vi "Handle Status Code.vi"(8 "error in":errorcluster, 10 "TPCANHandle":T1=81 items=["PCAN_NONEBUS"=0, "PCAN_USBBUS1"=81, "PCAN_USBBUS2"=82, "PCAN_USBBUS3"=83, "PCAN_USBBUS4"=84, "PCAN_USBBUS5"=85, "PCAN_USBBUS6"=86, "PCAN_USBBUS7"=87, "PCAN_USBBUS8"=88, "PCAN_USBBUS9"=1289, "PCAN_USBBUS10"=1290, "PCAN_USBBUS11"=1291, "PCAN_USBBUS12"=1292, "PCAN_USBBUS13"=1293, "PCAN_USBBUS14"=1294, "PCAN_USBBUS15"=1295, "PCAN_USBBUS16"=1296], 11 "TPCANStatus":T2 items=["PCAN_ERROR_OK"=0, "PCAN_ERROR_XMTFULL"=1, "PCAN_ERROR_OVERRUN"=2, "PCAN_ERROR_BUSLIGHT"=4, "PCAN_ERROR_BUSHEAVY"=8, "PCAN_ERROR_BUSPASSIVE"=262144, "PCAN_ERROR_BUSOFF"=16, "PCAN_ERROR_QRCVEMPTY"=32, "PCAN_ERROR_QOVERRUN"=64, "PCAN_ERROR_QXMTFULL"=128, "PCAN_ERROR_REGTEST"=256, "PCAN_ERROR_NODRIVER"=512, "PCAN_ERROR_HWINUSE"=1024, "PCAN_ERROR_NETINUSE"=2048, "PCAN_ERROR_ILLHW"=5120, "PCAN_ERROR_ILLNET"=6144, "PCAN_ERROR_ILLCLIENT"=7168, "PCAN_ERROR_RESOURCE"=8192, "PCAN_ERROR_ILLPARAMTYPE"=16384, "PCAN_ERROR_ILLPARAMVAL"=32768, "PCAN_ERROR_UNKNOWN"=65536, "PCAN_ERROR_ILLDATA"=131072, "PCAN_ERROR_ILLMODE"=524288, "PCAN_ERROR_CAUTION"=33554432, "PCAN_ERROR_INITIALIZE"=67108864, "PCAN_ERROR_ILLOPERATION"=134217728]) -> (0 "error out":errorcluster)   [LabVIEW 2018, in "PCANBasic.lvlib"]
uses:
  PCANBasic.lvlib
  TPCANStatus.ctl
  TPCANHandle.ctl
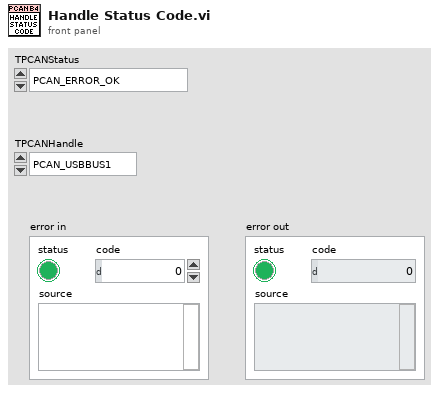
[diagram p1: front panel]
types:
  T1 = typedef "PCANBasic.lvlib/TPCANHandle.ctl" = u16
  T2 = typedef "PCANBasic.lvlib/TPCANStatus.ctl" = u32
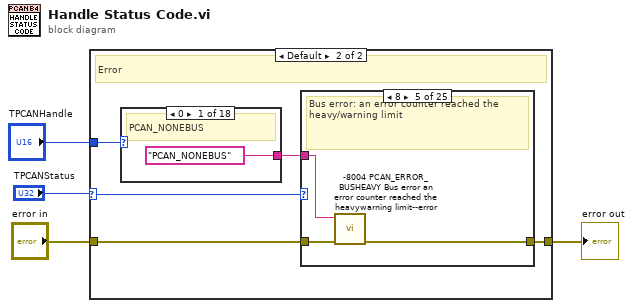
[diagram p0: block diagram]
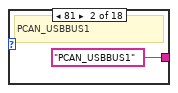
[diagram p3: hidden frame]
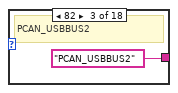
[diagram p4: hidden frame]
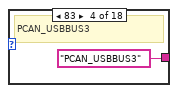
[diagram p5: hidden frame]
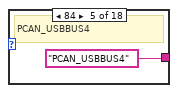
[diagram p6: hidden frame]
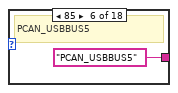
[diagram p7: hidden frame]
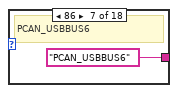
[diagram p8: hidden frame]
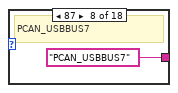
[diagram p9: hidden frame]
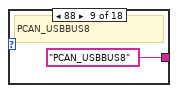
[diagram p10: hidden frame]
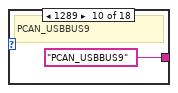
[diagram p11: hidden frame]
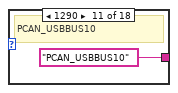
[diagram p12: hidden frame]
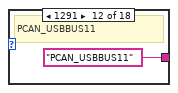
[diagram p13: hidden frame]
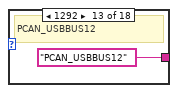
[diagram p14: hidden frame]
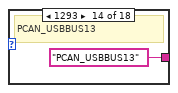
[diagram p15: hidden frame]
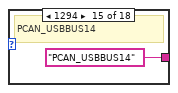
[diagram p16: hidden frame]
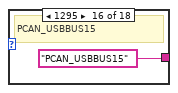
[diagram p17: hidden frame]
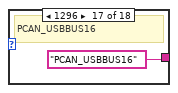
[diagram p18: hidden frame]
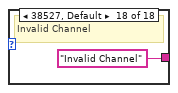
[diagram p19: hidden frame]
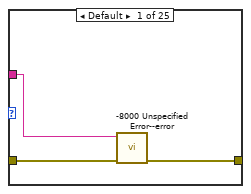
[diagram p20: hidden frame]
diagram:
  n1 = case shown="Default" "TPCANStatus" {
    selector: "TPCANStatus" -> [_ w10]
    tunnel: [w5 w8] -> w4
    tunnel: "error in" -> [w5 w9]
    tunnel: "TPCANHandle" -> [_ w7]
    frame 0 {
      # "OK"
    }
    frame Default {
      # "Error"
      n2 = case shown="0" w7 {
        tunnel: ["PCAN_NONEBUS" "PCAN_USBBUS1" "PCAN_USBBUS2" "PCAN_USBBUS3" "PCAN_USBBUS4" "PCAN_USBBUS5" "PCAN_USBBUS6" "PCAN_USBBUS7" "PCAN_USBBUS8" "PCAN_USBBUS9" "PCAN_USBBUS10" "PCAN_USBBUS11" "PCAN_USBBUS12" "PCAN_USBBUS13" "PCAN_USBBUS14" "PCAN_USBBUS15" "PCAN_USBBUS16" "Invalid Channel"] -> w6
        frame 0 {
          # "PCAN_NONEBUS"
        }
        frame 81 {
          # "PCAN_USBBUS1"
        }
        frame 82 {
          # "PCAN_USBBUS2"
        }
        frame 83 {
          # "PCAN_USBBUS3"
        }
        frame 84 {
          # "PCAN_USBBUS4"
        }
        frame 85 {
          # "PCAN_USBBUS5"
        }
        frame 86 {
          # "PCAN_USBBUS6"
        }
        frame 87 {
          # "PCAN_USBBUS7"
        }
        frame 88 {
          # "PCAN_USBBUS8"
        }
        frame 1289 {
          # "PCAN_USBBUS9"
        }
        frame 1290 {
          # "PCAN_USBBUS10"
        }
        frame 1291 {
          # "PCAN_USBBUS11"
        }
        frame 1292 {
          # "PCAN_USBBUS12"
        }
        frame 1293 {
          # "PCAN_USBBUS13"
        }
        frame 1294 {
          # "PCAN_USBBUS14"
        }
        frame 1295 {
          # "PCAN_USBBUS15"
        }
        frame 1296 {
          # "PCAN_USBBUS16"
        }
        frame 38527, Default {
          # "Invalid Channel"
        }
      }
      n3 = case shown="8" w10 {
        tunnel: w9 -> [w31 w34 w37 w40 w43 w46 w49 w52 w55 w58 w61 w64 w67 w70 w73 w76 w79 w82 w85 w88 w91 w94 w96 w100 w103]
        tunnel: [w30 w33 w36 w39 w42 w45 w48 w51 w54 w57 w60 w63 w66 w69 w72 w75 w78 w81 w84 w87 w90 w93 w97 w99 w102] -> w8
        tunnel: w6 -> [w29 w32 w35 w38 w41 w44 w47 w50 w53 w56 w59 w62 w65 w68 w71 w74 w77 w80 w83 w86 w89 w92 w95 w98 w101]
        frame Default {
          n4 = call "-8000 Unspecified Error--error.vi"("error in"=w31, "Argument"=w29) -> ("error out"=w30:errorcluster)  [unwired: 8 in, 1 out]
        }
        frame 1 {
          # "Transmit buffer in CAN controller is full"
          n5 = call "-8001 PCAN_ERROR_XMTFULL Transmit buffer in CAN controller is full--error.vi"("error in"=w34, "Channel"=w32) -> ("error out"=w33:errorcluster)  [unwired: 8 in, 1 out]
        }
        frame 2 {
          # "CAN Controller was read too late"
          n6 = call "-8002 PCAN_ERROR_OVERRUN CAN Controller was read too late--error.vi"("error in"=w37, "Channel"=w35) -> ("error out"=w36:errorcluster)  [unwired: 8 in, 1 out]
        }
        frame 4 {
          # "Bus error: an error counter reached the 'light' limit"
          n7 = call "-8003 PCAN_ERROR_BUSLIGHT Bus error an error counter reached the 'light' limit--error.vi"("error in"=w40, "Channel"=w38) -> ("error out"=w39:errorcluster)  [unwired: 8 in, 1 out]
        }
        frame 8 {
          # "Bus error: an error counter reached the heavy/warning limit"
          n8 = call "-8004 PCAN_ERROR_BUSHEAVY Bus error an error counter reached the heavywarning limit--error.vi"("error in"=w43, "Channel"=w41) -> ("error out"=w42:errorcluster)  [unwired: 8 in, 1 out]
        }
        frame 16 {
          # "Bus error: the CAN controller is in bus-off state"
          n9 = call "-8005 PCAN_ERROR_BUSOFF Bus error the CAN controller is in bus-off state--error.vi"("error in"=w46, "Channel"=w44) -> ("error out"=w45:errorcluster)  [unwired: 8 in, 1 out]
        }
        frame 32 {
          # "Receive queue is empty"
          n10 = call "-8006 PCAN_ERROR_QRCVEMPTY Receive queue is empty--error.vi"("error in"=w49, "Channel"=w47) -> ("error out"=w48:errorcluster)  [unwired: 8 in, 1 out]
        }
        frame 64 {
          # "Receive queue was read too late"
          n11 = call "-8024 PCAN_ERROR_QOVERRUN Receive queue was read too late--error.vi"("error in"=w52, "Channel"=w50) -> ("error out"=w51:errorcluster)  [unwired: 8 in, 1 out]
        }
        frame 128 {
          # "Transmit queue is full"
          n12 = call "-8007 PCAN_ERROR_QXMTFULL Transmit queue is full--error.vi"("error in"=w55, "Channel"=w53) -> ("error out"=w54:errorcluster)  [unwired: 8 in, 1 out]
        }
        frame 256 {
          # "Test of the CAN controller hardware registers failed (no hardware found)"
          n13 = call "-8008 PCAN_ERROR_REGTEST Test of the CAN controller hardware registers failed (no hardware found)--error.vi"("error in"=w58, "Channel"=w56) -> ("error out"=w57:errorcluster)  [unwired: 8 in, 1 out]
        }
        frame 512 {
          # "Driver not loaded"
          n14 = call "-8009 PCAN_ERROR_NODRIVER Driver not loaded--error.vi"("error in"=w61, "Channel"=w59) -> ("error out"=w60:errorcluster)  [unwired: 8 in, 1 out]
        }
        frame 1024 {
          # "Hardware already in use by a Net"
          n15 = call "-8010 PCAN_ERROR_HWINUSE Hardware already in use by a Net--error.vi"("error in"=w64, "Channel"=w62) -> ("error out"=w63:errorcluster)  [unwired: 8 in, 1 out]
        }
        frame 2048 {
          # "A Client is already connected to the Net"
          n16 = call "-8011 PCAN_ERROR_NETINUSE A Client is already connected to the Net--error.vi"("error in"=w67, "Channel"=w65) -> ("error out"=w66:errorcluster)  [unwired: 8 in, 1 out]
        }
        frame 6144 {
          # "Net handle is invalid"
          n17 = call "-8012 PCAN_ERROR_ILLHW Net handle is invalid--error.vi"("error in"=w70, "Channel"=w68) -> ("error out"=w69:errorcluster)  [unwired: 8 in, 1 out]
        }
        frame 6145 {
          # "Client handle is invalid"
          n18 = call "-8013 PCAN_ERROR_ILLCLIENT Client handle is invalid--error.vi"("error in"=w73, "Channel"=w71) -> ("error out"=w72:errorcluster)  [unwired: 8 in, 1 out]
        }
        frame 8192 {
          # "Resource (FIFO, Client, timeout) cannot be created"
          n19 = call "-8014 PCAN_ERROR_RESOURCE Resource (FIFO, Client, timeout) cannot be created--error.vi"("error in"=w76, "Argument"=w74) -> ("error out"=w75:errorcluster)  [unwired: 8 in, 1 out]
        }
        frame 16384 {
          # "Invalid parameter"
          n20 = call "-8015 PCAN_ERROR_ILLPARAMTYPE Invalid parameter--error.vi"("error in"=w79, "Channel"=w77) -> ("error out"=w78:errorcluster)  [unwired: 8 in, 1 out]
        }
        frame 32768 {
          # "Invalid parameter value"
          n21 = call "-8016 PCAN_ERROR_ILLPARAMVAL Invalid parameter value--error.vi"("error in"=w82, "Channel"=w80) -> ("error out"=w81:errorcluster)  [unwired: 8 in, 1 out]
        }
        frame 65536 {
          # "Unknown error"
          n22 = call "-8017 PCAN_ERROR_UNKNOWN Unknown error--error.vi"("error in"=w85, "Channel"=w83) -> ("error out"=w84:errorcluster)  [unwired: 8 in, 1 out]
        }
        frame 131072 {
          # "Invalid data, function, or action"
          n23 = call "-8018 PCAN_ERROR_ILLDATA Invalid data, function, or action--error.vi"("error in"=w88, "Channel"=w86) -> ("error out"=w87:errorcluster)  [unwired: 8 in, 1 out]
        }
        frame 524288 {
          # "Driver object state is wrong for the attempted operation"
          n24 = call "-8019 PCAN_ERROR_ILLMODE Driver object state is wrong for the attempted operation--error.vi"("error in"=w91, "Channel"=w89) -> ("error out"=w90:errorcluster)  [unwired: 8 in, 1 out]
        }
        frame 33554432 {
          # "An operation was successfully carried out, however, irregularities were registered"
          n25 = call "-8020 PCAN_ERROR_CAUTION An operation was successfully carried out, however, irregularities were registered--error.vi"("error in"=w94, "Channel"=w92) -> ("error out"=w93:errorcluster)  [unwired: 8 in, 1 out]
        }
        frame 67108864 {
          # "Channel is not initialized [Value was changed from 0x40000 to 0x4000000]"
          n26 = call "-8022 PCAN_ERROR_INITIALIZE Channel is not initialized--error.vi"("error in"=w96, "Channel"=w95) -> ("error out"=w97:errorcluster)  [unwired: 8 in, 1 out]
        }
        frame 134217728 {
          # "Invalid operation [Value was changed from 0x80000 to 0x8000000]"
          n27 = call "-8021 PCAN_ERROR_ILLOPERATION PCAN Invalid operation [Value was changed from 0x80000 to 0x8000000]--error.vi"("error in"=w100, "Channel"=w98) -> ("error out"=w99:errorcluster)  [unwired: 8 in, 1 out]
        }
        frame 262144 {
          # "Bus error: the CAN controller is error passive"
          n28 = call "-8023 PCAN_ERROR_ANYBUSERR Bus error the CAN controller is error passive--error.vi"("error in"=w103, "Channel"=w101) -> ("error out"=w102:errorcluster)  [unwired: 8 in, 1 out]
        }
      }
    }
  }
  "error out" <- w4
